vi "Read Dwell Time.vi"(8 "error in (no error)":errorcluster, 11 "Reader.lvclass in":refnum<class "Reader.lvclass">) -> (0 "error out":errorcluster, 1 "Classname":string, 2 "Dwell Time":dbl[unit], 3 "Reader.lvclass out":refnum<class "Reader.lvclass">)   [LabVIEW 2009, in "Reader.lvclass"]
doc: "Return the pre-set dwell time inside this Reader instance."
uses:
  Reader.lvclass
  Reader.lvclass/Reader.ctl
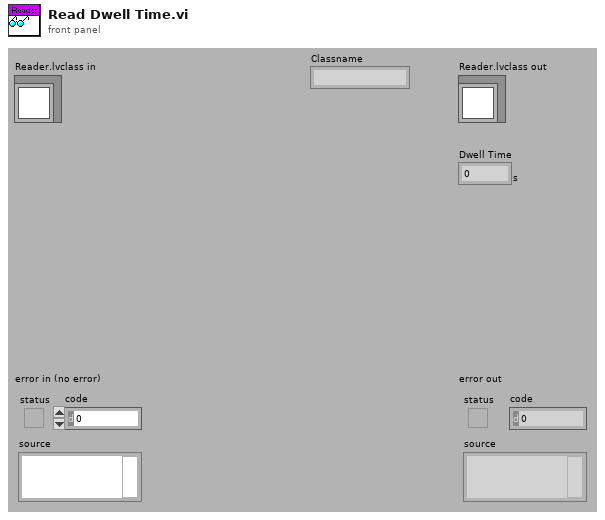
[diagram p1: front panel]
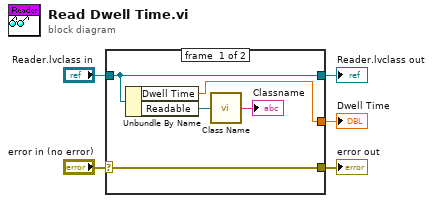
[diagram p0: block diagram]
diagram:
  n1 = case shown="No Error" "error in (no error)" {
    selector: "error in (no error)" -> [w10 w11]
    tunnel: [w10 w11] -> w4
    tunnel: [w9 w12] -> w2
    tunnel: "Reader.lvclass in" -> [w9 w12]
    tunnel: [w8 _] -> w1
    frame #0 {
      n2 = Unbundle By Name(w9) -> ("Dwell Time"=w8:dbl[unit], "Readable"=w7:refnum<class "Readable.lvclass">)
      n3 = call "Class Name.vi"("LabVIEW Object"=w7) -> ("Classname"=→"Classname":string)
    }
    frame #1 {
    }
  }
  "error out" <- w4
  "Reader.lvclass out" <- w2
  "Dwell Time" <- w1
